vi "IBM4_Diff_Read(VN).vi"(7 "Number":i32=10 min=1, 8 "error in":errorcluster, 9 "Neg-Chan":enum16{"A2", "A3", "A4", "A5"}(ring)=enum."A3", 10 "Pos-Chan":enum16{"A2", "A3", "A4", "A5"}(ring), 11 "COM resource in":refnum<visa-resource-name>="COM9") -> (0 "error out":errorcluster, 2 "array":dbl[](array[numeric]), 3 "COM resource out":refnum<visa-resource-name>)   [LabVIEW 2023, in "IBM4.lvlib"]
doc: "This VI interfaces with the IBM4 to perform a differential read operation.\n\nTshe number of readings should be greater than zero. At some point the number of reading will be too high and will cause a timeout error. This should only happen for numbers larger than 10000. The output will be an array of floating point (Voltage) values.\n\nAlternate read operations exist covering binary or floating point, single reading, multiple readings, and an average of multiple readings (floating point only)."
uses:
  <instrlib>/IBM4/IBM4.lvlib
  <vilib>/Instr/_visa.llb/VISA Configure Serial Port (Instr).vi
  <vilib>/regexp/Match Regular Expression.xnode
panel:
  out "error out 2":errorcluster
  out "read buffer":string
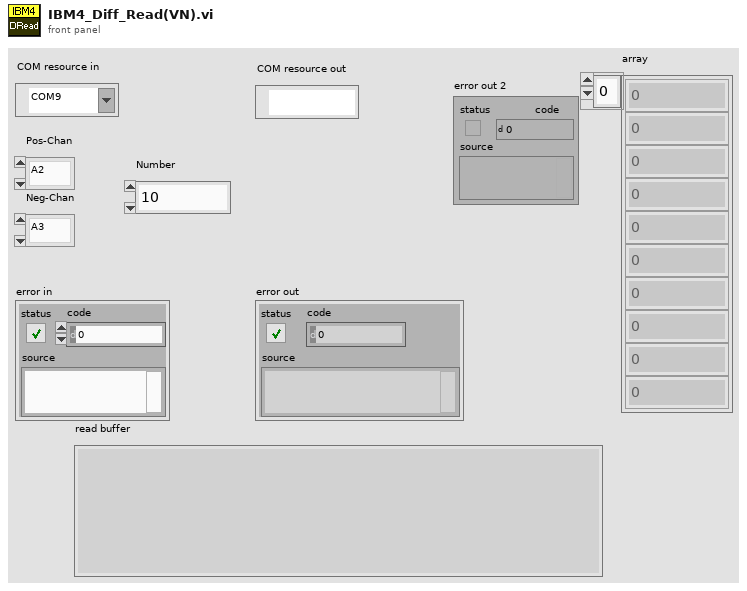
[diagram p1: front panel]
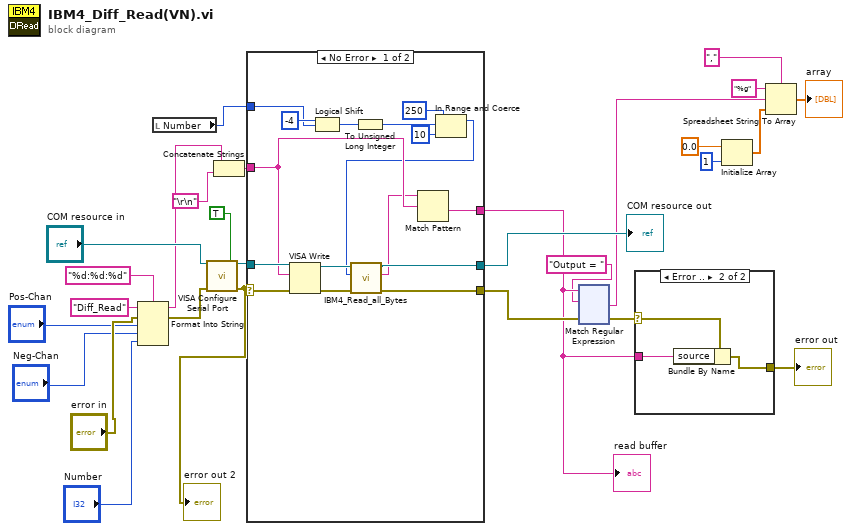
[diagram p0: block diagram]
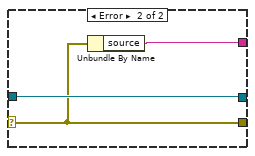
[diagram p3: hidden frame]
diagram:
  n1 = Format Into String(format string="%d:%d:%d", initial string="Diff_Read", error in="error in", "Pos-Chan", "Neg-Chan", "Number") -> (resulting string=w18:string, error out=w25:errorcluster)
  n2 = local read "Number"() -> (w3:i32)
  n3 = call-poly "VISA Configure Serial Port"("VISA resource name"="COM resource in", "Enable Termination\nChar (T)"=TRUE ("Enable Termination\nChar (T)"), "error in (no error)"=w25) -> ("VISA resource name out"=w22:refnum<visa-resource-name>, "error out"=w21:errorcluster)  [unwired: 11 in]
  "error out 2" <- w21
  n4 = Concatenate Strings(w18, "\r\n") -> (w17:string)
  n5 = case shown="No Error" w21 {
    selector: w21 -> [w41 w45]
    tunnel: w22 -> [w44 w47]
    tunnel: [w37 w45] -> w8
    tunnel: [w43 w46] -> w6
    tunnel: w17 -> [w42 _]
    tunnel: [w38 w47] -> w20
    tunnel: w3 -> [w30 _]
    frame No Error {
      n6 = VISA Write(VISA resource name=w44, write buffer=w42, error in (no error)=w41) -> (VISA resource name out=w40:refnum<visa-resource-name>, error out=w39:errorcluster)  [unwired: 1 out]
      n7 = Logical Shift(y=i16 -4, x=w30) -> (x << y=w33:i32)
      n8 = To Unsigned Long Integer(number=w33) -> (unsigned 32bit integer=w31:u32)
      n9 = In Range and Coerce(upper limit=u32 250, x=w31, lower limit=u32 10) -> (coerced(x)=w29:u32)  [unwired: 1 out]
      n10 = call <instrlib>:"IBM4_Read_all_Bytes.vi"("error in (no error)"=w39, "milliseconds to wait"=w29, "VISA Refnum in"=w40) -> ("error out"=w37:errorcluster, "String"=w36:string, "VISA Refnum out"=w38:refnum<visa-resource-name>)  [unwired: 2 in]
      n11 = Match Pattern(string=w36, regular expression=w42) -> (after substring=w43:string)  [unwired: 1 in, 3 out]
    }
    frame Error {
      n12 = Unbundle By Name(w45) -> ("source"=w46:string)
    }
  }
  "COM resource out" <- w20
  "read buffer" <- w6
  n13 = xnode "Match Regular Expression"("input string"=w6, "regular expression"="Output = " ("format string"), "error in"=w8) -> ("after match"=w4:string, "error out"=w7:errorcluster)  [unwired: 3 in, 3 out]
  n14 = case shown="Error .." w7 {
    selector: w7 -> [w48 w51]
    tunnel: [w48 w49] -> w16
    tunnel: w6 -> [_ w50]
    frame No Error {
    }
    frame Error {
      n15 = Bundle By Name(cluster=w51, "source"=w50) -> (w49:errorcluster)
    }
  }
  "error out" <- w16
  n16 = Initialize Array(0.0, 1 ("dimension size")) -> (w13:dbl[])
  n17 = Spreadsheet String To Array(delimiter (Tab)=",", format string="%g", spreadsheet string=w4, array type (2D Dbl)=w13) -> (array=→"array":dbl[])
